vi "SimpleAnyPackUnpack.vi"() -> ()   [LabVIEW 2019]
uses:
  <vilib>/gRPC/LabVIEW gRPC Library/Server API/typeDefs/Message Metadata.ctl
  <vilib>/gRPC/LabVIEW gRPC Library/Server API/typeDefs/Message Element Metadata.ctl
  <vilib>/gRPC/LabVIEW gRPC Library/Server API/typeDefs/Message Element Type.ctl
  54a96ed6-7513-4bf9-bbdc-367978e46fe7.vi
  63a71f1e-49c8-49e3-8f82-dda0691c2451.vi
  <vilib>/gRPC/LabVIEW gRPC Library/Server API/Server/Get Server DLL Path.vi
  <vilib>/gRPC/LabVIEW gRPC Library/gprc-lvsupport-release.lvlib
panel:
  out "error out":errorcluster
  out "Numeric":i32
  out "x = y?":bool
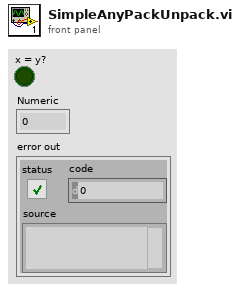
[diagram p1: front panel]
types:
  T1 = typedef "gprc-lvsupport-release.lvlib/Message Metadata.ctl" = cluster{"Version":i32, "Name":string, "Type Url":string, "Elements":T2[]}
  T2 = typedef "gprc-lvsupport-release.lvlib/Message Element Metadata.ctl" = cluster{"Embedded Message Name":string, "Protobuf Index":i32, "MessageElementType":T3, "Repeated":bool}
  T3 = typedef "gprc-lvsupport-release.lvlib/Message Element Type.ctl" = enum32{"Int32Value", "FloatValue", "DoubleValue", "BoolValue", "StringValue", "MessageValue", "Int64Value", "UInt32Value", "UInt64Value", "EnumValue", "Bytes", "Fixed64", "Fixed32", "SFixed64", "SFixed32", "SInt64", "SInt32"}
  T4 = typedef "gprc-lvsupport-release.lvlib/grpcId.ctl" = u64
  T5 = typedef "gprc-lvsupport-release.lvlib/Any.ctl" = cluster{"Type Url":string, "Bytes":u8[]}
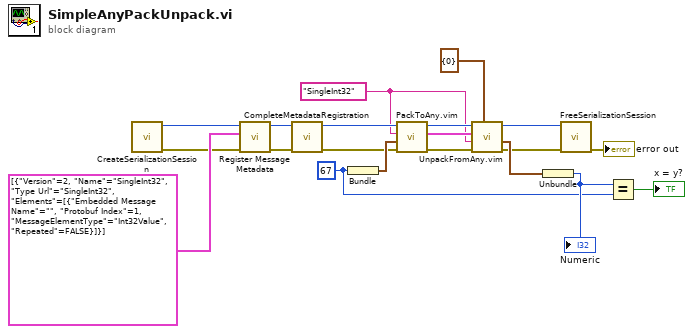
[diagram p0: block diagram]
diagram:
  w17 = 67
  w9 = "SingleInt32" ("Message Type")
  n1 = call <vilib>:"CreateSerializationSession.vi"() -> ("error out"=w6:errorcluster, "Serialization Session ID"=w20:T4)  [unwired: 10 in]
  n2 = call <vilib>:"Register Message Metadata.vi"("error in (no error)"=w6, "Messages"=T1[] [{"Version"=2, "Name"="SingleInt32", "Type Url"="SingleInt32", "Elements"=[{"Embedded Message Name"="", "Protobuf Index"=1, "MessageElementType"=enum."Int32Value", "Repeated"=FALSE}]}], "gRPCid"=w20) -> ("error out"=w5:errorcluster, "gRPCid"=w15:T4)  [unwired: 7 in]
  n3 = call <vilib>:"CompleteMetadataRegistration.vi"("error in (no error)"=w5, "gRPC ID"=w15) -> ("error out"=w4:errorcluster, "gRPC ID Out"=w14:T4)  [unwired: 8 in]
  n4 = Bundle(w17) -> (w13:cluster{i32})  [unwired: 1 in]
  n5 = call "PackToAny.vim"("error in (no error)"=w4, "Data To Pack"=w13, "Message Type"=w9, "gRPCid in"=w14) -> ("error out"=w3:errorcluster, "Any"=w10:T5, "gRPCid"=w12:u64)  [unwired: 5 in]
  n6 = call "UnpackFromAny.vim"("Data Type"=cluster{i32} {0}, "error in (no error)"=w3, "Message Type"=w9, "Any"=w10, "gRPCid in"=w12) -> ("error out"=w2:errorcluster, "Unpacked Value"=w8:cluster{i32}, "gRPCid"=w7:u64)  [unwired: 4 in]
  n7 = Unbundle(w8) -> (w18:i32)
  "Numeric" <- w18
  n8 = call <vilib>:"FreeSerializationSession.vi"("error in (no error)"=w2, "Serialization Session ID"=w7) -> ("error out"=→"error out":errorcluster)  [unwired: 9 in]
  n9 = Equal?(x=w18, y=w17) -> (x = y?=→"x = y?":bool)
